vi "1_MNIST_Model_Converter.vi"() -> ()   [LabVIEW 2020]
uses:
  <vilib>/Ngene/Deep Learning Toolkit/Toolkit/NN_Network/Controls/NN_Device.ctl
  <vilib>/Ngene/DeepLTK FPGA Addon/Toolkit/NNF_Host/Low_Level/Network_Converter/Controls/Range_Calculation_Specs.ctl
  <vilib>/Ngene/Deep Learning Toolkit/Toolkit/Deep_Learning_Toolkit_by_Ngene.lvlib
  <vilib>/Ngene/DeepLTK FPGA Addon/Toolkit/DeepLTK_FPGA_Addon.lvlib
panel:
  in  "Dataset Path":path
  out "error out":errorcluster
  in  "Wights file":path=path "D:/Ngene/GitHub/deepltk_fpga_examples/1_MNIST_Classification(PXI,sbRIO)/Models/0_Original/MNIST_CNN/MNIST_CNN_weights_24_11_25__15_33_35.bin"
  in  "Configuration file":path=path "D:/Ngene/GitHub/deepltk_fpga_examples/1_MNIST_Classification(PXI,sbRIO)/Models/0_Original/MNIST_CNN/MNIST_CNN_net_cfg_24_11_25__15_33_35.cfg"
  out "Generated_Files":path[](array[path])=[path "D:/Ngene/Projects_SVN/DeepLTK_FPGA/Projects/Examples/1_MNIST_Classification(PXI,sbRIO)/Models/1_Converted/mnist_cnn/NNF_mnist_cnn_net_cfg_24_11_25__15_36_06.cfg", path "D:/Ngene/Projects_SVN/DeepLTK_FPGA/Projects/Examples/1_MNIST_Classification(PXI,sbRIO)/Models/1_Converted/mnist_cnn/NNF_mnist_cnn_weights_24_11_25__15_36_06.bin", path "D:/Ngene/Projects_SVN/DeepLTK_FPGA/Projects/Examples/1_MNIST_Classification(PXI,sbRIO)/Models/1_Converted/mnist_cnn/NNF_mnist_cnn_render_24_11_25__15_36_06.svg", path "D:/Ngene/Projects_SVN/DeepLTK_FPGA/Projects/Examples/1_MNIST_Classification(PXI,sbRIO)/Models/1_Converted/mnist_cnn/NNF_mnist_cnn_net_scalers_24_11_25__15_36_06.cfg"]
  in  "Dest":path=path "D:/Ngene/GitHub/deepltk_fpga_examples/1_MNIST_Classification(PXI,sbRIO)/Models/1_Converted"
  # "Overview: This example demonstrates the preparation process of pretrained MNIST model to be deployed on FPGA.\nIt consists of the following stages:\n1. Network optimization by merging applicable layers together.\n2. Per layer weights and output statistics calculation for optimal quantization on FPGA.\n3. Saving converted model together with statistical information to be used during the deployment.\nRequirements:\n•DeepLTK - Deep Learning Toolkit for LabVIEW (https://www.ngene.co/deep-learning-toolkit-for-labview)\n•DeepLTK FPGA Addon(https://www.ngene.co/deepltk-accelerator-for-fpga)\n•Sample dataset for reliable output statistic calculation. \nInstructions: \n1.\tProvide the path to the configuration file of a pretrained model in the \"Configuration File\" control.\n2.\tProvide the path to the weights file of a pretrained model in the \"Weights File\" control. \n3.\tProvide the path to the MNIST dataset used during training in the \"Dataset Path\" control. \n4.\tProvide the destination directory where the results will be stored in the \"Dest\" control.\n5.\tRun the VI and wait until all processes are completed.\n\nThe resulting files (Scalers .cfg, Weights .bin, and Configuration .cfg) will be stored at paths displayed in \"Generated_Files\" indicator.\nThis files will be used during inference process.\nMore Examples: https://github.com/ngenehub/deepltk_fpga_examples"
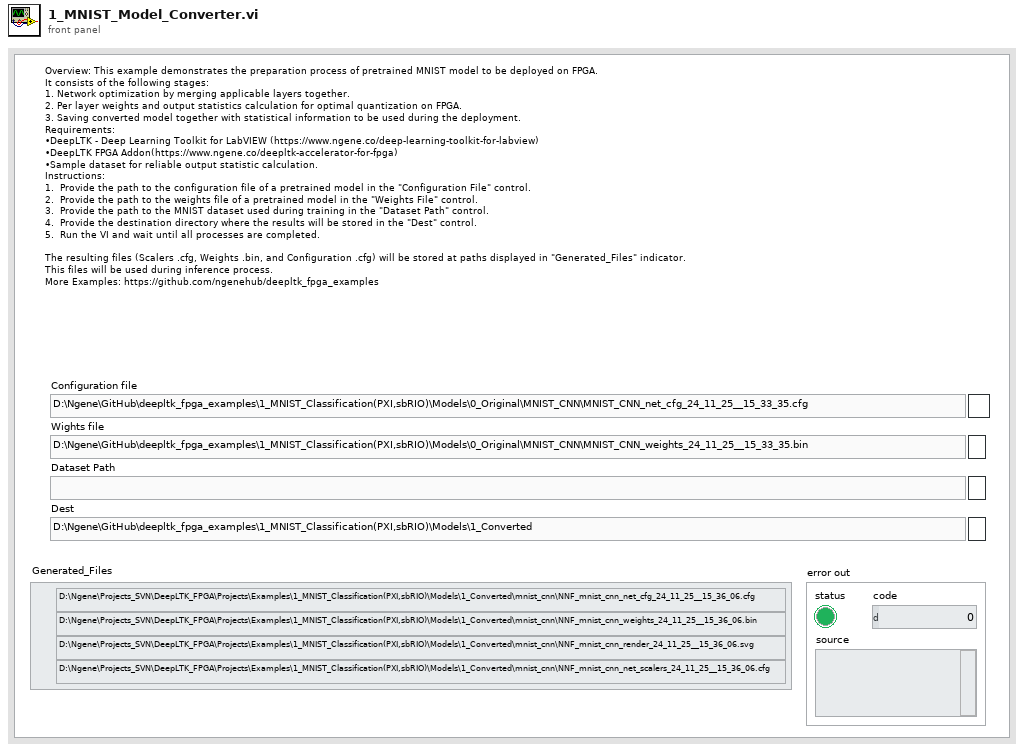
[diagram p1: front panel]
types:
  T1 = typedef "DeepLTK_FPGA_Addon.lvlib/Range_Calculation_Specs.ctl" = cluster{"# of Histogram Bins":i32, "Outputs Range Percentile(0.9999)":dbl, "Weights Range Percentile(0.9999)":dbl}
  T2 = typedef "Deep_Learning_Toolkit_by_Ngene.lvlib/NN_Device.ctl" = enum16{"CPU", "GPU"}
  T3 = typedef "Deep_Learning_Toolkit_by_Ngene.lvlib/NN_DataSets_All(In3D_Out1D).ctl" = cluster{"Train":T4, "Validation":T4, "Test":T4}
  T4 = typedef "Deep_Learning_Toolkit_by_Ngene.lvlib/NN_DataSet(In3D_Out1D).ctl" = cluster{"Inputs Ref.":variant, "Outputs Ref.":T5, "Dataset_Size":i32, "Dims_In":T6, "Dims_Out":i32, "Labels":string[], "File Paths":path[]}
  T5 = typedef "Deep_Learning_Toolkit_by_Ngene.lvlib/NN_Data_ref(2D_SGL).ctl" = refnum<data-value>
  T6 = typedef "Deep_Learning_Toolkit_by_Ngene.lvlib/NN_Dims(C,H,W).ctl" = cluster{"C":i32, "H":i32, "W":i32}
  T7 = typedef "Deep_Learning_Toolkit_by_Ngene.lvlib/NN_Config_Params.ctl" = cluster{"Name":string, "mBatch":i32, "NN_Train_Params":T8, "LR_Decay_Policy":T11, "Labels":string[], "Loss":T13}
  T8 = typedef "Deep_Learning_Toolkit_by_Ngene.lvlib/NN_Train_Params.ctl" = cluster{"Optimizer":T9, "Beta_1":sgl, "Beta_2":sgl, "Weight Decay(L1)":sgl, "Weight Decay(L2)":sgl, "Data_Sampling":T10}
  T9 = typedef "Deep_Learning_Toolkit_by_Ngene.lvlib/NN_Train_Optimizer.ctl" = enum16{"SGD", "Adam", "Adagrad", "Adadelta", "RMSProp", "Nesterov"}
  T10 = typedef "Deep_Learning_Toolkit_by_Ngene.lvlib/NN_Train_Data_Sampling.ctl" = enum16{"Random", "Sequential"}
  T11 = typedef "Deep_Learning_Toolkit_by_Ngene.lvlib/NN_LR_Policy_Cfg.ctl" = cluster{"Policy_Type":T12, "LR0":dbl, "k":sgl, "WarmUp_Policy":enum16{"Step", "Ramp"}, "WarmUp_Iter":i32, "WarmUp_Ratio":sgl}
  T12 = typedef "Deep_Learning_Toolkit_by_Ngene.lvlib/NN_LR_Policy_Type.ctl" = enum16{"Manual", "Step", "Exp", "1/t"}
  T13 = typedef "Deep_Learning_Toolkit_by_Ngene.lvlib/NN_Loss_Config_Params.ctl" = cluster{"Loss_Type":T14, "Loss_Conf_Params":variant}
  T14 = typedef "Deep_Learning_Toolkit_by_Ngene.lvlib/NN_Loss_Type.ctl" = enum16{"None", "MSE", "CrossEntropy", "YOLO_v2", "YOLO_v4"}
  T15 = typedef "Deep_Learning_Toolkit_by_Ngene.lvlib/NN_Layer_Config_Params.ctl" = cluster{"Layer_Type":T16, "Layer_Conf_Params":variant, "Input Layers":string[]}
  T16 = typedef "Deep_Learning_Toolkit_by_Ngene.lvlib/NN_Layer_Type.ctl" = enum16{"Input1D", "Input3D", "Conv1D", "Conv2D", "Conv2D_Adv", "MaxPool", "AvgPool", "UpSample", "DropOut3D", "ShortCut", "Concat", "SoftMax3D", "FC", "DropOut", "Softmax", "Flatten", "YOLO_v2", "YOLO_v4", "Activation", "BatchNormalization", "Unsupported"}
  T17 = typedef "Deep_Learning_Toolkit_by_Ngene.lvlib/NN.ctl" = cluster{"Name":string, "No of Layers":i32, "mBatch":i32, "Layers":T18[], "Dimty":T19, "Dims_In":T6, "Dims_Out":T6, "Working_Dir":path, "Train?":bool, "Train_Params":T8, "LR_Update_Policy":T11, "Session Data":T20, "Ground_truth":T21, "NNg_hdls":T22, "NN_Device":T2, "GPU Id":i32, "Labels":string[], "Receptive Field":T23[], "Loss_Type":T14, "Loss_Cfg_Prms":variant, "NNG_WS":T24}
  T18 = typedef "Deep_Learning_Toolkit_by_Ngene.lvlib/NN_Layer_ref.ctl" = refnum<data-value>
  T19 = typedef "Deep_Learning_Toolkit_by_Ngene.lvlib/NN_In_Out_Dim-ty.ctl" = enum8{"In1D_Out1D", "In3D_Out1D", "In3D_Out3D", "In3D_OutBBox"}
  T20 = typedef "Deep_Learning_Toolkit_by_Ngene.lvlib/NN_Train_Session_Data.ctl" = cluster{"Epochs":sgl, "Tot_Iter":i32, "LR":sgl, "LR_iter":i32}
  T21 = typedef "Deep_Learning_Toolkit_by_Ngene.lvlib/NN_Ground_truth.ctl" = cluster{"Y":variant}
  T22 = typedef "Deep_Learning_Toolkit_by_Ngene.lvlib/nng_cuda_handles.ctl" = cluster{"cudnn":u64, "cublas":u64, "stream":u64, "curand":u64}
  T23 = typedef "Deep_Learning_Toolkit_by_Ngene.lvlib/NN_Dims(V,H).ctl" = cluster{"V":i32, "H":i32}
  T24 = typedef "Deep_Learning_Toolkit_by_Ngene.lvlib/NNG_WS.ctl" = cluster{"NNG_WS_Mem":T25, "Max_WS_Size":i64}
  T25 = typedef "Deep_Learning_Toolkit_by_Ngene.lvlib/NNg_WS_Mem_DVR.ctl" = refnum<data-value>
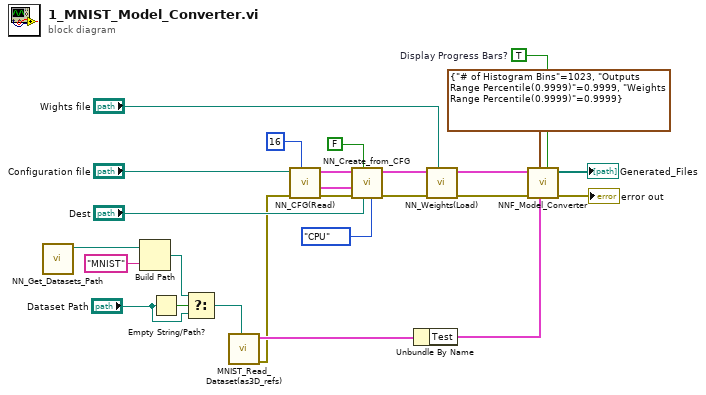
[diagram p0: block diagram]
diagram:
  w9 = TRUE  # Display Progress Bars?
  n1 = call "NN_Get_Datasets_Path.vi"() -> ("Datasets path"=w1:path)  [unwired: 11 in]
  n2 = Build Path(base path=w1, name or relative path="MNIST") -> (appended path=w7:path)
  n3 = Empty String/Path?(string/path="Dataset Path") -> (empty?=w6:bool)
  n4 = Select(t=w7, s=w6, f="Dataset Path") -> (s? t:f=w5:path)
  n5 = call "MNIST_Read_Dataset(as3D_refs).vi"("MNIST Dataset Path"=w5) -> ("error out"=w2:errorcluster, "Data(3D)_Refs"=w3:T3)  [unwired: 9 in]
  n6 = call <vilib>:"NN_CFG(Read).vi"("mBatch"=16, "error in (no error)"=w2, "CFG file path"="Configuration file") -> ("error out"=w23:errorcluster, "Net_Cfg"=w26:T7, "Layer_Cfg"=w22:T15[])  [unwired: 6 in]
  n7 = call <vilib>:"NN_Create_from_CFG.vi"("NN_Device"=NN_Device."CPU", "Working Dir"="Dest", "Train? (false)"=FALSE, "error in (no error)"=w23, "Net_Cfg"=w26, "Layer_Cfg"=w22) -> ("error out"=w24:errorcluster, "NN out"=w25:T17)  [unwired: 4 in]
  n8 = Unbundle By Name(w3) -> ("Test"=w15:T4)
  n9 = call <vilib>:"NN_Weights(Load).vi"("Weight File Path"="Wights file", "error in (no error)"=w24, "NN in"=w25) -> ("error out"=w18:errorcluster, "NN out"=w19:T17)  [unwired: 7 in]
  n10 = call <vilib>:"NNF_Model_Converter.vi"("Display Progress Bars?"=w9, "DataSet"=w15, "Range_Calculation_Specs"=T1 {"# of Histogram Bins"=1023, "Outputs Range Percentile(0.9999)"=0.9999, "Weights Range Percentile(0.9999)"=0.9999}, "error in (no error)"=w18, "NN in"=w19) -> ("error out"=→"error out":errorcluster, "Generated_Files"=→"Generated_Files":path[])  [unwired: 3 in, 2 out]
